vi "CreateNiceXMLString.vi"(11 "Top Node":refnum<k20>) -> (3 "XML String":string)   [LabVIEW 2017]
uses:
  <resource>/objmgr/DOMUserDefRef.rc
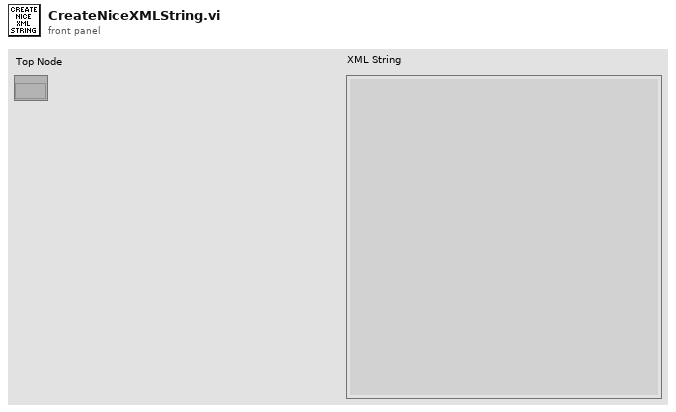
[diagram p1: front panel]
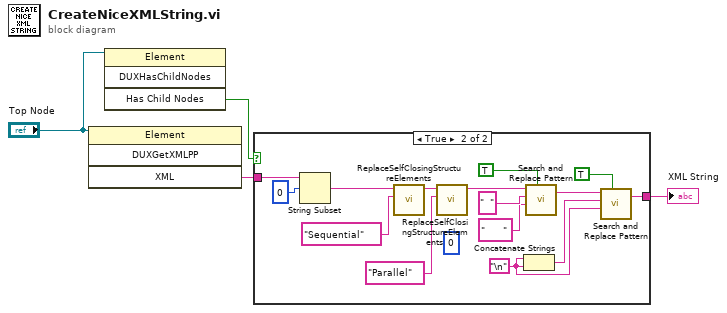
[diagram p0: block diagram]
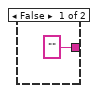
[diagram p2: hidden frame]
diagram:
  n1 = invoke class="Element" method="DUXGetXMLPP"(reference="Top Node") -> ("XML"=w1:string)  [unwired: 3 in, 3 out]
  n2 = invoke class="Element" method="DUXHasChildNodes"(reference="Top Node") -> ("Has Child Nodes"=w2:bool)  [unwired: 3 in, 3 out]
  n3 = case shown="True" w2 {
    tunnel: ["" ("result string") w17] -> w4
    tunnel: w1 -> [_ w11]
    frame False {
    }
    frame True {
      (unwired) 0
      w18 = "\n"
      n4 = String Subset(string=w11, offset (0)=0) -> (substring=w7:string)  [unwired: 1 in]
      n5 = call "ReplaceSelfClosingStructureElements.vi"("Replace String"="Sequential", "String In"=w7) -> ("String Out"=w6:string)  [unwired: 9 in]
      n6 = call "ReplaceSelfClosingStructureElements.vi"("Replace String"="Parallel", "String In"=w6) -> ("String Out"=w9:string)  [unwired: 9 in]
      n7 = Concatenate Strings(w18, w18) -> (w19:string)
      n8 = call <vilib>:"Search and Replace Pattern.vi"("string"=w9, "regular expression (\"\")"="  " ("regular expression (\"\")"), "replace string (\"\")"="      " ("regular expression (\"\")"), "replace all? (F)"=TRUE) -> ("result string"=w12:string)  [unwired: 1 in, 1 out]
      n9 = call <vilib>:"Search and Replace Pattern.vi"("string"=w12, "regular expression (\"\")"=w19, "replace string (\"\")"=w18, "replace all? (F)"=TRUE) -> ("result string"=w17:string)  [unwired: 1 in, 1 out]
    }
  }
  "XML String" <- w4
